vi "LightningPID.vi"(8 "PID Settings":T1, 9 "Reset":bool, 10 "Position":dbl, 11 "Set Point":dbl) -> (3 "Output":dbl)   [LabVIEW 2015]
uses:
  LightningPID Settings.ctl
panel:
  out "dBase":dbl(graph)
  out "iState":dbl(graph)
  out "dBase":dbl
  out "iState":dbl
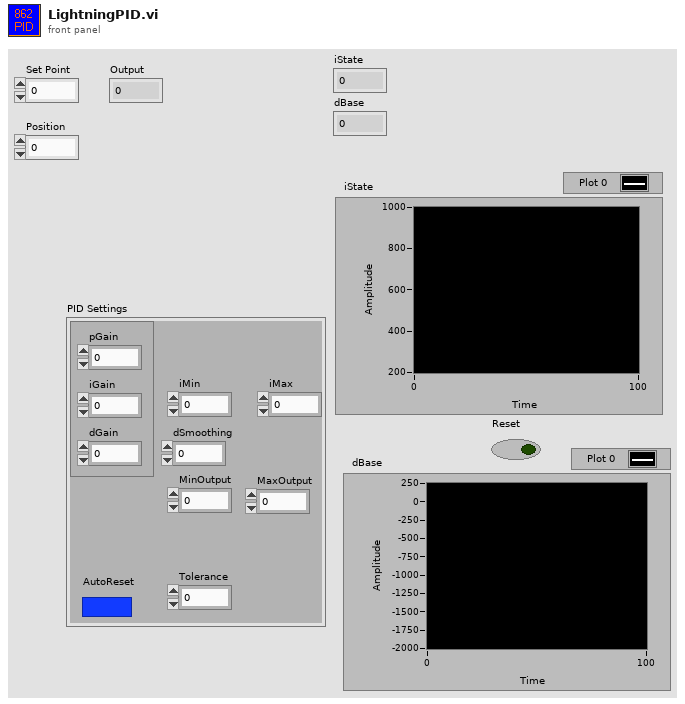
[diagram p1: front panel]
types:
  T1 = typedef "LightningPID Settings.ctl" = cluster{"iMax":dbl, "iMin":dbl, "iGain":dbl, "pGain":dbl, "dGain":dbl, "MaxOutput":dbl, "MinOutput":dbl, "AutoReset":bool, "Tolerance":dbl, "dSmoothing":dbl}
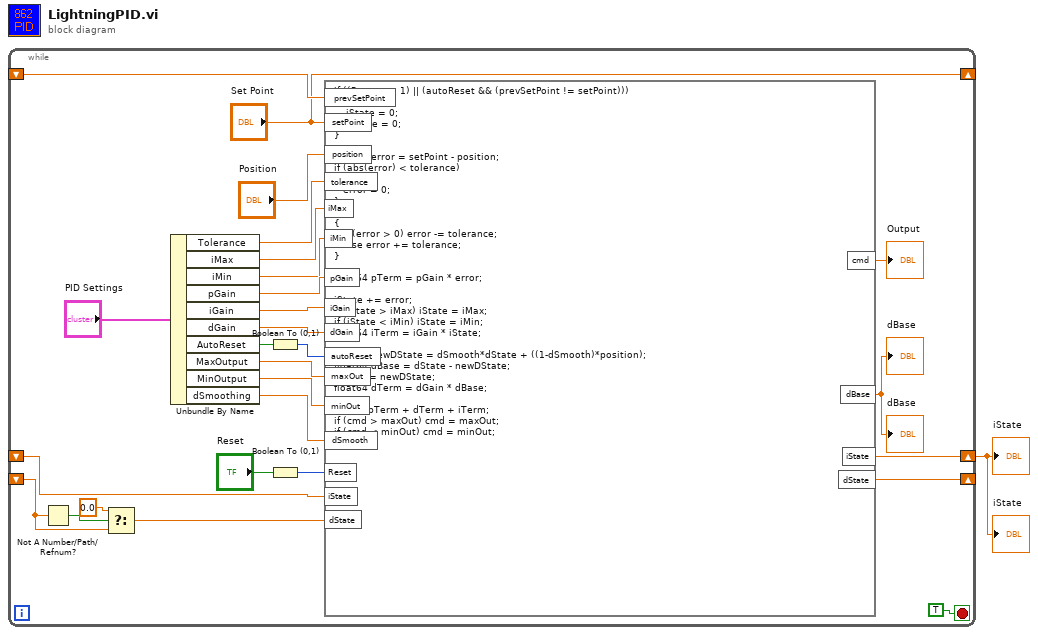
[diagram p0: block diagram]
diagram:
  n1 = while {
    shift-right: [w22] -> w1
    shift-left: _ -> [w20]
    shift-right: [w21] -> _
    shift-left: _ -> [w3]
    shift-right: ["Set Point"] -> _
    shift-left: _ -> [w19]
    stop <- TRUE stop-if-true
    n2 = Not A Number/Path/Refnum?(number/path/refnum=w3) -> (NaN/Path/Refnum?=w5:bool)
    n3 = Select(t=0.0, s=w5, f=w3) -> (s? t:f=w2:dbl)
    n4 = Unbundle By Name("PID Settings") -> ("Tolerance"=w8:dbl, "iMax"=w27:dbl, "iMin"=w10:dbl, "pGain"=w26:dbl, "iGain"=w25:dbl, "dGain"=w24:dbl, "AutoReset"=w17:bool, "MaxOutput"=w12:dbl, "MinOutput"=w11:dbl, "dSmoothing"=w7:dbl)
    n5 = Boolean To (0,1)(Boolean=w17) -> (0, 1=w18:i16)
    n6 = Boolean To (0,1)(Boolean="Reset") -> (0, 1=w16:i16)
    n7 = formula code="if ((Reset == 1) || (autoReset && (prevSetPoint != setPoint)))\n{\n    iState = 0;\n    dState = 0;\n}\n\nfloat64 error = setPoint - position;\nif (abs(error) < tolerance) \n{\n   error = 0;\n}\nelse\n{\n   if (error > 0) error -= tolerance;\n   else error += tolerance;\n}\n\nfloat64 pTerm = pGain * error;\n\niState += error;\nif (iState > iMax) iState = iMax;\nif (iState < iMin) iState = iMin;\nfloat64 iTerm = iGain * iState;\n\nfloat64 newDState = dSmooth*dState + ((1-dSmooth)*position);\nfloat64 dBase = dState - newDState;\ndState = newDState;\nfloat64 dTerm = dGain * dBase;\n\ncmd = pTerm + dTerm + iTerm;\nif (cmd > maxOut) cmd = maxOut;\nif (cmd < minOut) cmd = minOut;"("position"="Position", "dState"=w2, "iState"=w20, "pGain"=w26, "iGain"=w25, "dGain"=w24, "iMax"=w27, "iMin"=w10, "Reset"=w16, "prevSetPoint"=w19, "autoReset"=w18, "setPoint"="Set Point", "maxOut"=w12, "minOut"=w11, "tolerance"=w8, "dSmooth"=w7) -> ("cmd"=→"Output":dbl, "iState"=w22:dbl, "dState"=w21:dbl, "dBase"=→"dBase" →"dBase":dbl)
  }
  "iState" <- w1
  "iState" <- w1
